vi "Shorten Type Name.vi"(11 "Name In":string) -> (3 "Limited Name":string)   [LabVIEW 2020, in "Better Search.lvlib" / "BetterSearch.lvclass"]
uses:
  BetterSearch.lvclass
  <vilib>/regexp/Match Regular Expression.xnode
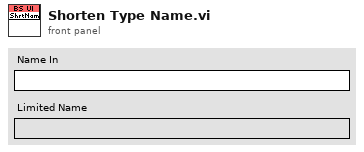
[diagram p1: front panel]
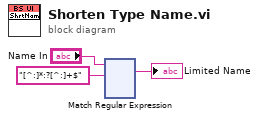
[diagram p0: block diagram]
diagram:
  n1 = xnode "Match Regular Expression"("input string"="Name In", "regular expression"="[^:]*:?[^:]+$") -> ("whole match"=→"Limited Name":string)  [unwired: 4 in, 4 out]
